vi "getWavelength_v80AM2.vi"() -> ()   [LabVIEW 2016]
uses:
  x32/CLDevIFace.dll
panel:
  in  "Clear Chart?":bool
  in  "Delay Time (s)":dbl=0.01
  out "XY Graph":cluster{i32[], dbl[]}(graph)
  out "error out":errorcluster
  out "output param":i32
  in  "stop":bool
  in  "OK Button":bool
  out "Wavelength":dbl format="%.9f"
  in  "CommPort":dbl=5.0 caption="Comm Port #"
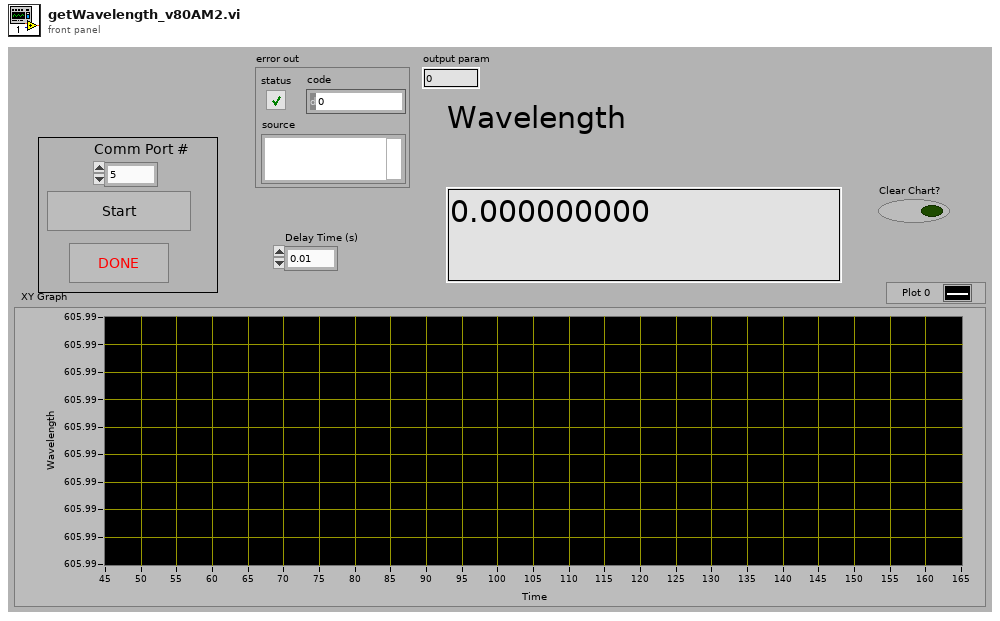
[diagram p1: front panel]
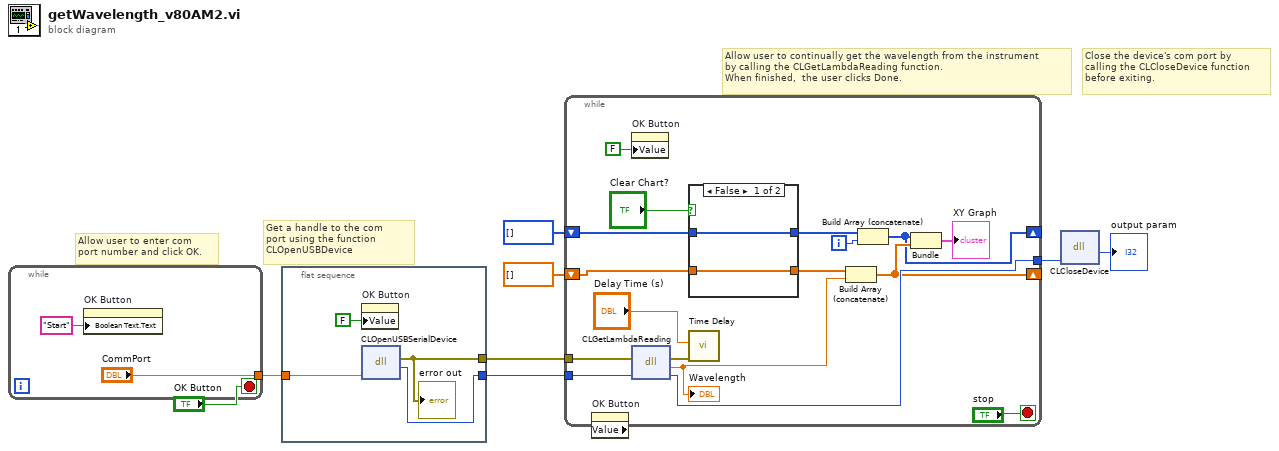
[diagram p0: block diagram]
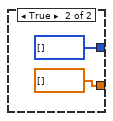
[diagram p2: hidden frame]
diagram:
  # "Close the device's com port by\ncalling the CLCloseDevice function\nbefore exiting."
  # "Allow user to continually get the wavelength from the instrument\nby calling the CLGetLambdaReading function.  \nWhen finished,  the user clicks Done."
  # "Get a handle to the com\nport using the function CLOpenUSBDevice"
  # "Allow user to enter com \nport number and click OK."
  n1 = while {
    tunnel: ["CommPort"] -> w7
    stop <- "OK Button" stop-if-true
    n2 = property on="OK Button" class="Bool (strict)"("Boolean Text.Text"="Start") -> ()  [unwired: 2 in, 2 out]
  }
  n3 = flat-sequence {
    tunnel: w7 -> [w14]
    tunnel: [w13] -> w6
    tunnel: [w11] -> w1
    frame #0 {
      n4 = property on="OK Button" class="Bool (strict)"("Value"=FALSE) -> ()  [unwired: 2 in, 2 out]
      n5 = dll-call lib="C:/Users/Lab/Desktop/Bristol wavemeter 621/00424-2-00 621 customer CD/Programming Interface/x32/CLDevIface.dll" fn="CLOpenUSBSerialDevice"("commPort"=w14) -> (error out=w11:errorcluster, "return type"=w13:i32)  [unwired: 4 in, 1 out]
      "error out" <- w11
    }
  }
  n6 = while {
    tunnel: w6 -> [w31]
    tunnel: [w29] -> w5
    shift-right: [w25] -> _
    shift-left: dbl[] [] -> [w19]
    shift-right: [w24] -> _
    shift-left: i32[] [] -> [w18]
    tunnel: w1 -> [w20]
    i -> [w28]
    stop <- "stop" stop-if-true
    n7 = property on="OK Button" class="Bool (strict)" props=["Value"]() -> ()  [unwired: 2 in, 3 out]
    n8 = property on="OK Button" class="Bool (strict)"("Value"=FALSE) -> ()  [unwired: 2 in, 2 out]
    n9 = dll-call lib="C:/Users/Lab/Desktop/Bristol wavemeter 621/00424-2-00 621 customer CD/Programming Interface/x32/CLDevIface.dll" fn="CLGetLambdaReading"(error in=w20, "devHandle"=w31) -> (error out=w21:errorcluster, "return type"=w27:dbl, "devHandle"=w29:i32)  [unwired: 2 in, 1 out]
    "Wavelength" <- w27
    n10 = case shown="False" "Clear Chart?" {
      tunnel: w19 -> [w32 _]
      tunnel: w18 -> [w33 _]
      tunnel: [w33 i32[] []] -> w16
      tunnel: [w32 dbl[] []] -> w15
      frame False {
      }
      frame True {
      }
    }
    n11 = call "Time Delay"("error in (no error)"=w21, "Delay Time (s)"="Delay Time (s)") -> ()  [unwired: 9 in, 1 out]
    n12 = Build Array (concatenate)(w15, w27) -> (w25:dbl[])
    n13 = Build Array (concatenate)(w16, w28) -> (w24:i32[])
    n14 = Bundle(w24, w25) -> (→"XY Graph":cluster{i32[], dbl[]})  [unwired: 1 in]
  }
  n15 = dll-call lib="C:/Users/Lab/Desktop/Bristol wavemeter 621/00424-2-00 621 customer CD/Programming Interface/x32/CLDevIface.dll" fn="CLCloseDevice"("commPort"=w5) -> ("return type"=→"output param":i32)  [unwired: 4 in, 2 out]
